vi "Read Multi.vi"(0 "tdms file in":refnum<k34>, 5 "group":string, 7 "Channel":string[](array[string]), 9 "Numeric":dbl, 11 "error in (no error)":errorcluster) -> (4 "tdms file out":refnum<k34>, 6 "Array":dbl[][](array[numeric]), 10 "Length":u64, 15 "error out":errorcluster)   [LabVIEW 2013, in "MFC.LVLIB" / "MFC.lvclass"]
uses:
  MFC.lvclass
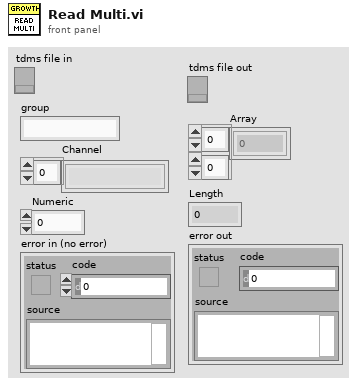
[diagram p1: front panel]
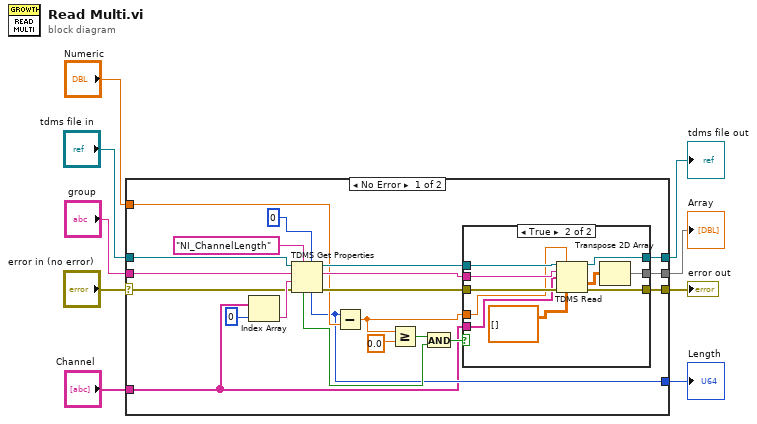
[diagram p0: block diagram]
diagram:
  n1 = case shown="No Error" "error in (no error)" {
    selector: "error in (no error)" -> [w10 w43]
    tunnel: "tdms file in" -> [w11 w44]
    tunnel: "group" -> [w30 _]
    tunnel: "Channel" -> [w15 _]
    tunnel: [w13 w44] -> w1
    tunnel: [w12 w43] -> w7
    tunnel: "Numeric" -> [w24 _]
    tunnel: [w14 _] -> w6
    tunnel: [w18 _] -> w5
    frame No Error {
      n2 = Index Array(array=w15, index=0) -> (element=w16:string)
      n3 = TDMS Get Properties(5:u64 0, 7:"NI_ChannelLength" ("channel name(s) in"), 8:w10, 9:w16, 10:w30, 11:w11) -> (0:w27:errorcluster, 2:w25:string, 3:w26:refnum<k34>, 4:w18:u64, 6:w22:bool)  [unwired: 1 out]
      n4 = Subtract(x=w18, y=w24) -> (x-y=w21:dbl)
      n5 = Greater Or Equal?(x=w21, y=0.0) -> (x >= y?=w19:bool)
      n6 = And(x=w19, y=w22) -> (x .and. y?=w23:bool)
      n7 = case shown="True" w23 {
        tunnel: [w31 w42] -> w12
        tunnel: [w32 w41] -> w13
        tunnel: w27 -> [w31 w40]
        tunnel: w26 -> [w32 w39]
        tunnel: w25 -> [_ w38]
        tunnel: w15 -> [_ w37]
        tunnel: w21 -> [_ w35]
        tunnel: [_ w33] -> w14
        frame False {
        }
        frame True {
          n8 = TDMS Read(0:w39, 1:w35, 5:w38, 7:w37, 11:w40, 12:dbl[][] []) -> (4:w41:refnum<k34>, 10:w34:dbl[][], 15:w42:errorcluster)  [unwired: 2 in, 3 out]
          n9 = Transpose 2D Array(2D array=w34) -> (transposed array=w33:dbl[][])
        }
      }
    }
    frame Error {
    }
  }
  "error out" <- w7
  "Length" <- w5
  "Array" <- w6
  "tdms file out" <- w1
